vi "Untitled 8.vi"() -> ()   [LabVIEW 2018, in "Tests.lvlib" / "Compile.lvlib"]
uses:
  Compile.lvlib
  src/Toolkit/Low-Level/Context/Compiler.lvclass
  src/Toolkit/Low-Level/Lexer/Lexer.lvclass
  src/Toolkit/Low-Level/Readers/String/String.lvclass
  D:/Users/cfield/Code/Field R&D Services/Labstache/src/Toolkit/Low-Level/Readers/Reader/Reader.lvclass
  src/Toolkit/Data/Datum/Datum.lvclass
panel:
  in  "Data":refnum<class "Datum.lvclass">
  in  "Value":string
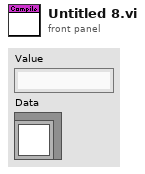
[diagram p1: front panel]
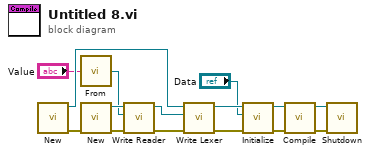
[diagram p0: block diagram]
diagram:
  n1 = call "New.vi"() -> ("Error Out"=w13:errorcluster, "Compiler"=w10:refnum<class "Compiler.lvclass">)  [unwired: 10 in]
  n2 = call "From.vi"("Value"="Value") -> ("String"=w9:refnum<class "String.lvclass">)
  n3 = call "New.vi"("Error In"=w13) -> ("Error Out"=w14:errorcluster, "Lexer"=w15:refnum<class "Lexer.lvclass">)  [unwired: 9 in]
  n4 = call-dynamic "Write Reader.vi"("Error In"=w14, "Reader"=w9, "Lexer In"=w15) -> ("Error Out"=w12:errorcluster, "Lexer Out"=w11:refnum<class "Lexer.lvclass">)  [unwired: 7 in]
  n5 = call-dynamic "Write Lexer.vi"("Error In"=w12, "Lexer"=w11, "Compiler In"=w10) -> ("Error Out"=w6:errorcluster, "Compiler Out"=w7:refnum<class "Compiler.lvclass">)  [unwired: 7 in]
  n6 = call-dynamic "Initialize.vi"("Error In"=w6, "Data"="Data", "Compiler In"=w7) -> ("Error Out"=w3:errorcluster, "Compiler Out"=w4:refnum<class "Compiler.lvclass">)  [unwired: 7 in]
  n7 = call-dynamic "Compile.vi"("Error In"=w3, "Compiler In"=w4) -> ("Error Out"=w1:errorcluster, "Compiler Out"=w2:refnum<class "Compiler.lvclass">)  [unwired: 8 in]
  n8 = call "Shutdown.vi"("Error In"=w1, "Context In"=w2) -> ()  [unwired: 7 in, 3 out]
